vi "VisionV3 2-7-20.vi"(7 "error in":errorcluster, 10 "Image In":T2) -> (0 "error out":errorcluster, 1 "Number of Matches":i32, 2 "Shape Report":T1(array[cluster]) {"Score" format="%.2f"; "Centroid"."y" format="%.2f"; "Centroid"."x" format="%.2f"}, 3 "Image Out":T2)   [LabVIEW 2019]
uses:
  <vilib>/vision/Image Controls.llb/IMAQ Image.ctl
  <vilib>/vision/NI_Vision_Development_Module.lvlib
panel:
  out "Histogram (Histogram 1)":u32[][](array[numeric])
  out "Histogram Graph":u32[][](graph)
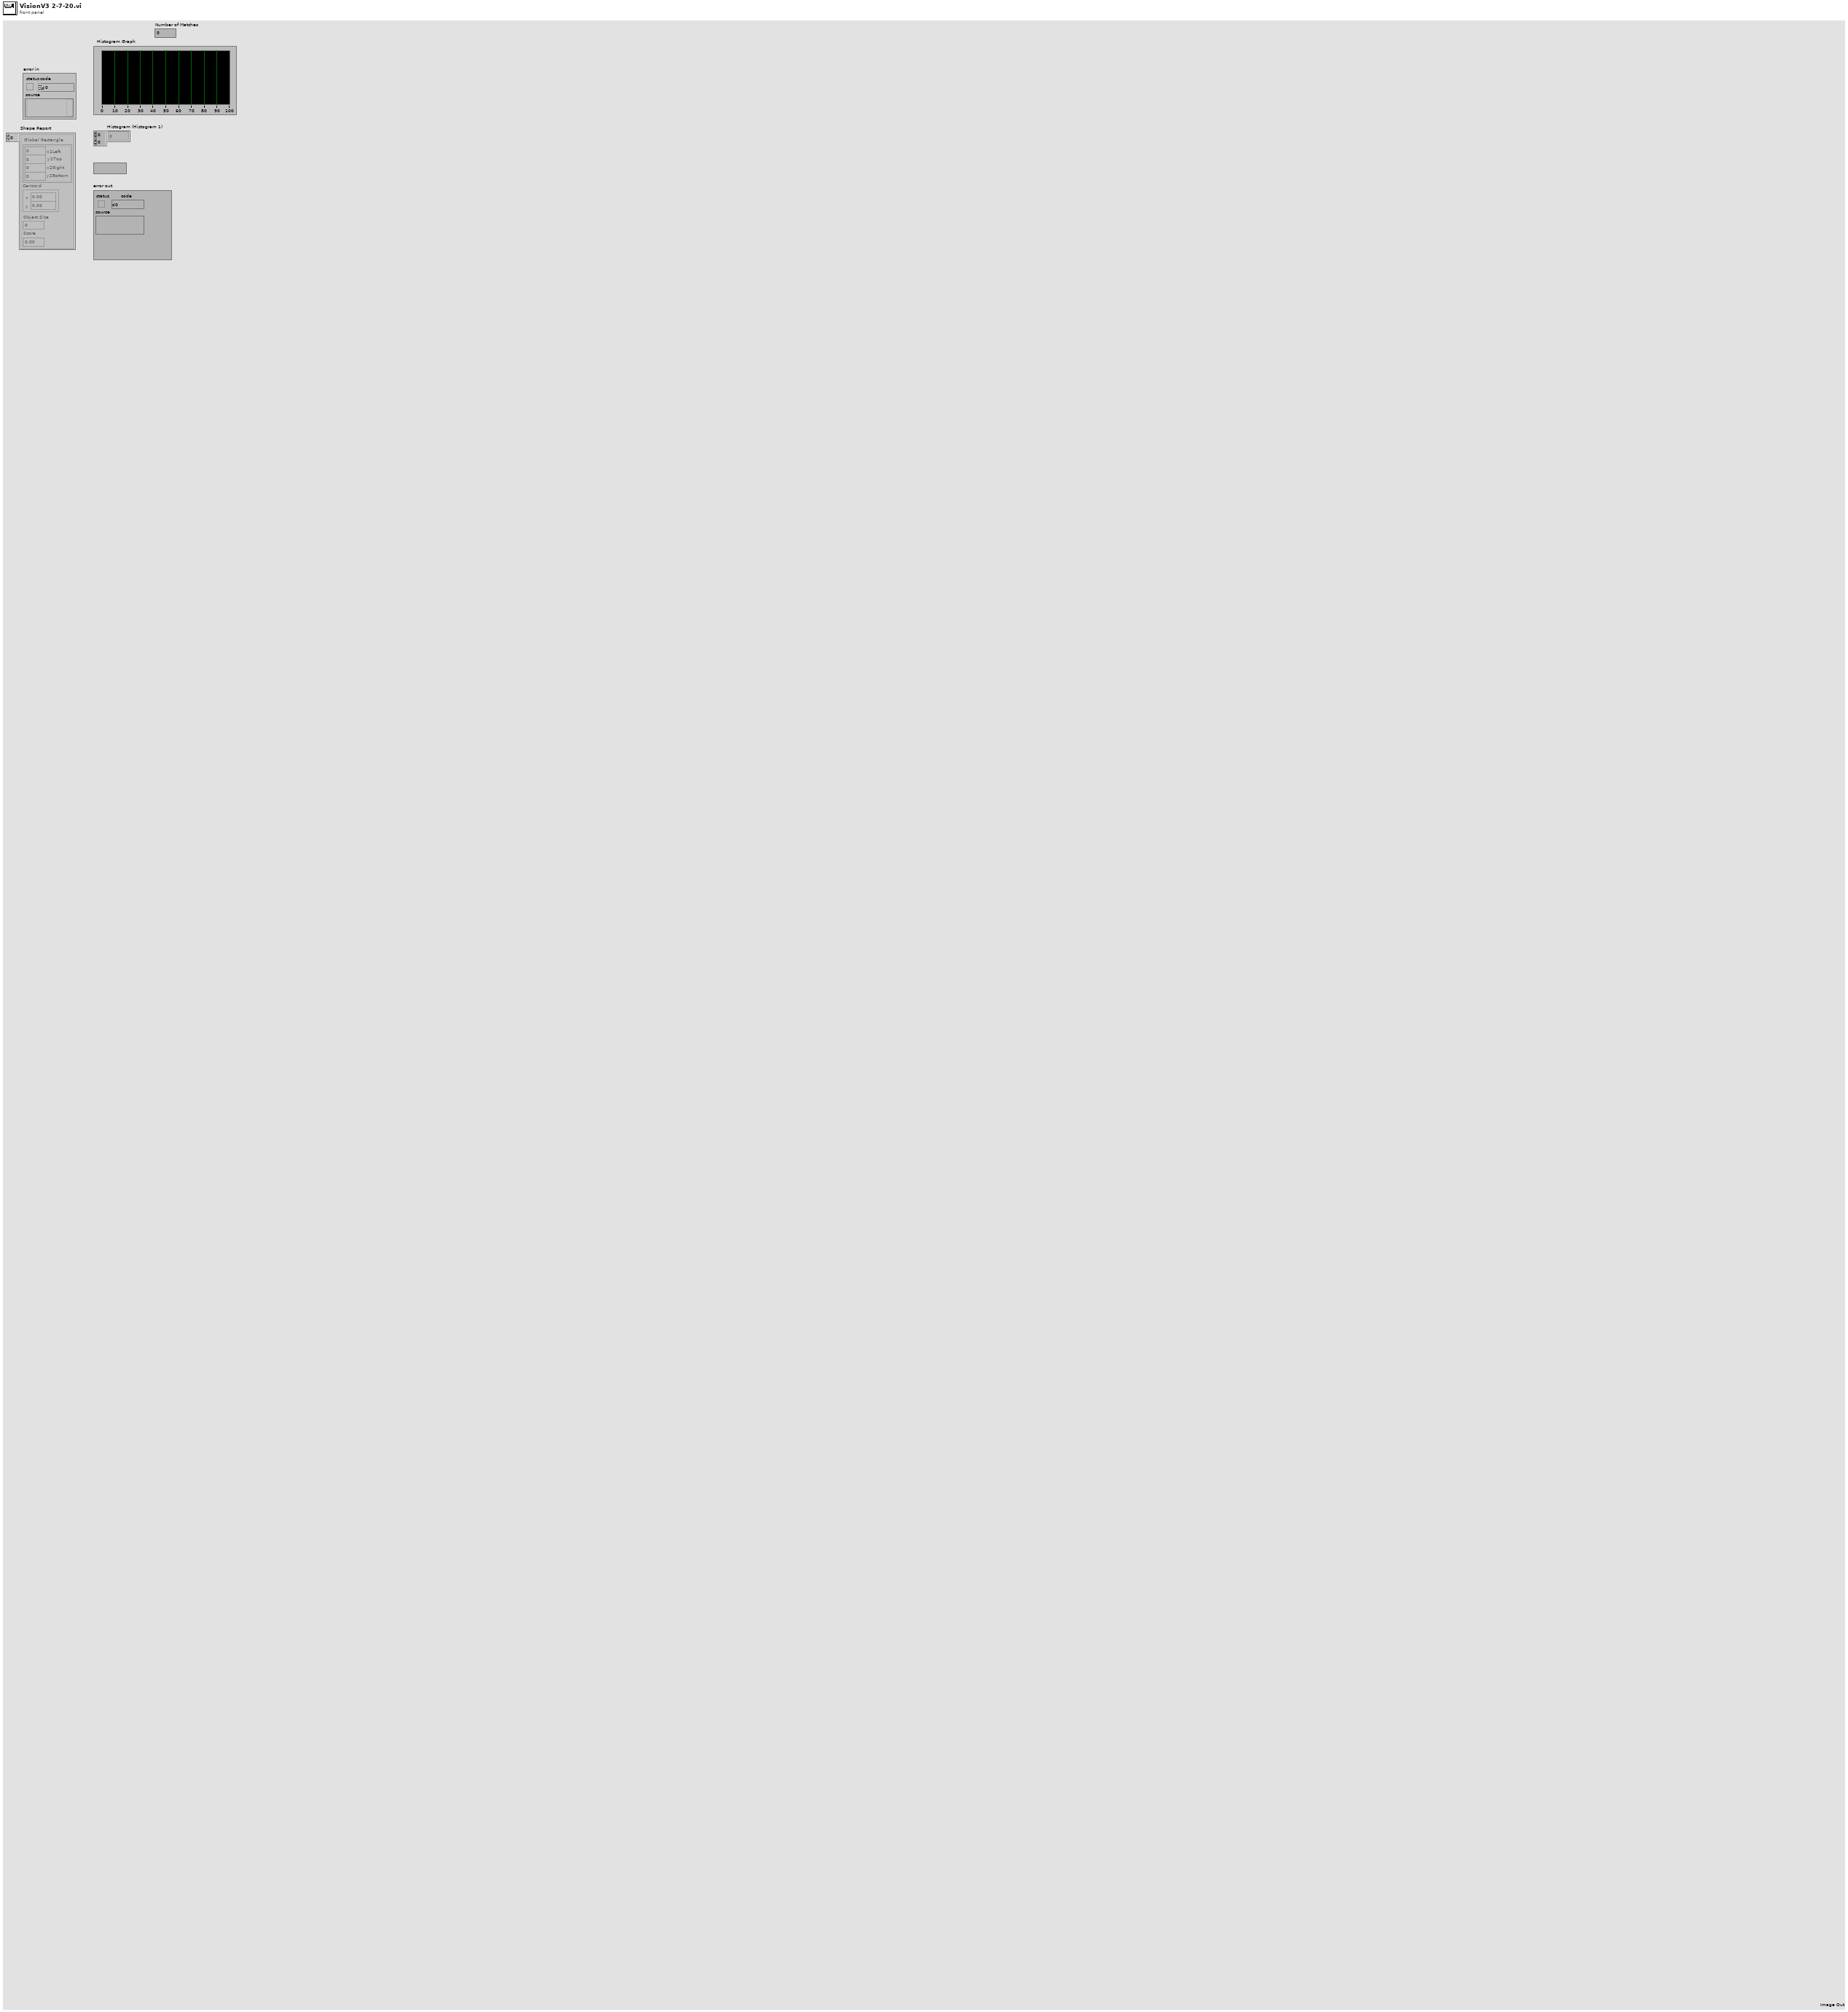
[diagram p1: front panel]
types:
  T1 = cluster{"Global Rectangle":cluster{"x1Left":i32, "y1Top":i32, "x2Right":i32, "y2Bottom":i32}, "Centroid":cluster{"x":sgl, "y":sgl}, "Object Size":u32, "Score":dbl}[]
  T2 = typedef "IMAQ Image.ctl" = refnum<image>
  T3 = enum32{"AutoM", "Close", "Dilate", "Erode", "Gradient", "Gradient in", "Gradient out", "HitMiss", "Open", "PClose", "POpen", "Thick", "Thin"}
  T4 = cluster{"Global Rectangle":i32[], "Contours":cluster{"ID":enum32{"External", "Internal"}, "Type":u32, "Coordinates":i32[]}[]}
  T5 = cluster{"histogram":u32[], "Minimal Value":sgl, "Maximal Value":sgl, "Starting Value":sgl, "Interval Width":sgl, "Mean Value":sgl, "Standard  Variation":sgl, "Area (pixels)":i32}
  T6 = typedef "Image Type" = u32
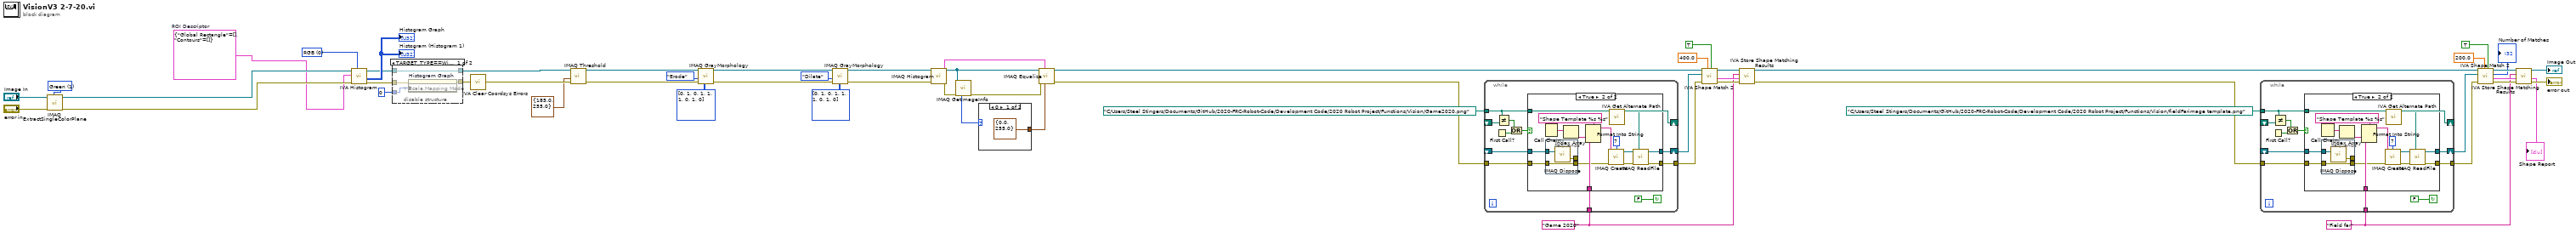
[diagram p0: block diagram]
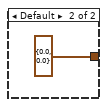
[diagram p4: hidden frame]
diagram:
  w2 = "Field far" ("Step Name")
  w14 = "Game 2020" ("Step Name")
  w49 = u16 0 items=["RGB", "HSL", "HSV", "HSI"] ("Color Mode")
  w47 = T4 {"Global Rectangle"=[], "Contours"=[]}  # ROI Descriptor
  w55 = 1 items=["Red", "Green", "Blue", "Hue", "Saturation", "Luminance", "Value", "Intensity"] ("Color Plane")
  n1 = call "IMAQ ExtractSingleColorPlane"("Color Plane"=w55, "error in (no error)"="error in", "Image Src"="Image In") -> ("error out"=w52:errorcluster, "Image Dst Out"=w51:T2)  [unwired: 1 in, 6 out]
  n2 = call <vilib>:"IVA Histogram.vi"("Color Mode"=w49, "error in (no error)"=w52, "ROI Descriptor"=w47, "Image In"=w51) -> ("error out"=w50:errorcluster, "Histograms"=→"Histogram Graph" →"Histogram (Histogram 1)":u32[][], "Image Out"=w46:T2)  [unwired: 5 out]
  n3 = disable-structure "Conditional Disable Structure" shown="TARGET_TYPE==Windows" {
    disable-tunnel: w50 -> [w59 w60]
    disable-tunnel: [w58 w60] -> w44
    disable-tunnel: w46 -> [w57 w61]
    disable-tunnel: [w57 w61] -> w41
    disable-tunnel: u8 0 ("Y Scale.Mapping Mode") -> [w56 _]
    frame condition #0 {
      n4 = property on="Histogram Graph" class="WFGraph (strict)"(error in=w59, "Y Scale.Mapping Mode"=w56) -> (error out=w58:errorcluster)  [unwired: 1 in, 1 out]
    }
    frame condition #1 (active) {
    }
  }
  n5 = call <vilib>:"IVA Clear Coordsys Errors.vi"("error in (no error)"=w44) -> ("error out"=w43:errorcluster)  [unwired: 10 in]
  n6 = call "IMAQ Threshold"("error in (no error)"=w43, "Range"=cluster{"Lower value":sgl, "Upper value":sgl} {"Lower value"=185.0, "Upper value"=255.0}, "Image Src"=w41) -> ("error out"=w40:errorcluster, "Image Dst Out"=w37:T2)  [unwired: 3 in, 4 out]
  n7 = call "IMAQ GrayMorphology"("Structuring Element"=i32[][] [[0, 1, 0], [1, 1, 1], [0, 1, 0]], "error in (no error)"=w40, "Operation"=T3."Erode", "Image Src"=w37) -> ("error out"=w36:errorcluster, "Image Dst Out"=w33:T2)  [unwired: 3 in, 3 out]
  n8 = call "IMAQ GrayMorphology"("Structuring Element"=i32[][] [[0, 1, 0], [1, 1, 1], [0, 1, 0]], "error in (no error)"=w36, "Operation"=T3."Dilate", "Image Src"=w33) -> ("error out"=w32:errorcluster, "Image Dst Out"=w28:T2)  [unwired: 3 in, 3 out]
  n9 = call "IMAQ Histogram"("error in (no error)"=w32, "Image"=w28) -> ("error out"=w27:errorcluster, "Histogram Report"=w30:T5)  [unwired: 3 in, 5 out]
  n10 = call "IMAQ GetImageInfo"("error in (no error)"=w27, "Image"=w28) -> ("error out"=w26:errorcluster, "Image Type"=w29:T6)  [unwired: 8 out]
  n11 = case shown="0" w29 {
    tunnel: [cluster{"Minimum":sgl, "Maximum":sgl} {"Minimum"=0.0, "Maximum"=255.0} ("Range") cluster{"Minimum":sgl, "Maximum":sgl} {"Minimum"=0.0, "Maximum"=0.0} ("Range")] -> w25
    frame 0 {
    }
    frame Default {
    }
  }
  n12 = call "IMAQ Equalize"("Range"=w25, "Histogram Report"=w30, "error in (no error)"=w26, "Image Src"=w28) -> ("error out"=w31:errorcluster, "Image Dst Out"=w22:T2)  [unwired: 2 in, 4 out]
  n13 = while {
    shift-right: [w74] -> w15
    shift-left: _ -> [w73]
    tunnel: [w71] -> w16
    tunnel: w31 -> [w70]
    tunnel: path "C:/Users/Steel Stingers/Documents/GitHub/2020-FRC-Robot-Code/Development Code/2020 Robot Project/Functions/Vision/Game2020.png" ("Template Path") -> [w68]
    tunnel: w14 -> [w69]
    shift-right: [w68] -> _
    shift-left: _ -> [w67]
    stop <- FALSE continue-if-true
    n14 = First Call?() -> (First Call?: T/F=w66:bool)
    n15 = Not Equal?(x=w68, y=w67) -> (x != y?=w65:bool)
    n16 = Or(x=w65, y=w66) -> (x .or. y?=w64:bool)
    n17 = case shown="True" w64 {
      tunnel: [w76 w88] -> w74
      tunnel: w73 -> [w76 w79]
      tunnel: [w75 w86] -> w71
      tunnel: w70 -> [w75 w78]
      tunnel: w68 -> [_ w81]
      tunnel: w69 -> [_ w82]
      frame False {
      }
      frame True {
        n18 = Call Chain() -> (call chain=w84:string[])
        n19 = stacked-sequence {
          tunnel: w79 -> [w94]
          tunnel: w78 -> [w93]
          tunnel: [w93] -> w77
          tunnel: [w92] -> _
          frame #0 {
            n20 = call "IMAQ Dispose"("Image"=w94) -> ("error out"=w92:errorcluster)  [unwired: 2 in, 3 out]
          }
        }
        n21 = Index Array(array=w84) -> (element=w83:string)  [unwired: 1 in]
        n22 = Format Into String(format string="Shape Template %s %s" ("Image Name"), w83, w82) -> (resulting string=w91:string)  [unwired: 2 in, 1 out]
        n23 = call "IMAQ Create"("Border Size"=7, "Image Name"=w91, "error in (no error)"=w77) -> ("New Image"=w89:T2, "error out"=w87:errorcluster)  [unwired: 1 in, 1 out]
        n24 = call <vilib>:"IVA Get Alternate Path.vi"("Path In"=w81) -> ("Path Out"=w80:path)  [unwired: 10 out]
        n25 = call "IMAQ ReadFile"("File Path"=w80, "error in (no error)"=w87, "Image"=w89) -> ("error out"=w86:errorcluster, "Image Out"=w88:T2)  [unwired: 2 in, 5 out]
      }
    }
  }
  n26 = call <vilib>:"IVA Shape Match 2.vi"("Scale Invariance"=TRUE, "Minimal Score"=400.0, "error in (no error)"=w16, "Template"=w15, "Image Src"=w22) -> ("error out"=w21:errorcluster, "Shape Report"=w19:T1, "Image Out"=w18:T2)  [unwired: 4 out]
  n27 = call <vilib>:"IVA Store Shape Matching Results.vi"("error in (no error)"=w21, "Shape Report"=w19, "Step Name"=w14, "Image in"=w18) -> ("error out"=w20:errorcluster, "Image dup"=w11:T2)  [unwired: 6 out]
  n28 = while {
    shift-right: [w105] -> w3
    shift-left: _ -> [w104]
    tunnel: [w102] -> w4
    tunnel: w20 -> [w101]
    tunnel: path "C:/Users/Steel Stingers/Documents/GitHub/2020-FRC-Robot-Code/Development Code/2020 Robot Project/Functions/Vision/fieldFarimage template.png" ("Template Path") -> [w99]
    tunnel: w2 -> [w100]
    shift-right: [w99] -> _
    shift-left: _ -> [w98]
    stop <- FALSE continue-if-true
    n29 = First Call?() -> (First Call?: T/F=w97:bool)
    n30 = Not Equal?(x=w99, y=w98) -> (x != y?=w96:bool)
    n31 = Or(x=w96, y=w97) -> (x .or. y?=w95:bool)
    n32 = case shown="True" w95 {
      tunnel: [w107 w119] -> w105
      tunnel: w104 -> [w107 w110]
      tunnel: [w106 w117] -> w102
      tunnel: w101 -> [w106 w109]
      tunnel: w99 -> [_ w112]
      tunnel: w100 -> [_ w113]
      frame False {
      }
      frame True {
        n33 = Call Chain() -> (call chain=w115:string[])
        n34 = stacked-sequence {
          tunnel: w110 -> [w125]
          tunnel: w109 -> [w124]
          tunnel: [w124] -> w108
          tunnel: [w123] -> _
          frame #0 {
            n35 = call "IMAQ Dispose"("Image"=w125) -> ("error out"=w123:errorcluster)  [unwired: 2 in, 3 out]
          }
        }
        n36 = Index Array(array=w115) -> (element=w114:string)  [unwired: 1 in]
        n37 = Format Into String(format string="Shape Template %s %s" ("Image Name"), w114, w113) -> (resulting string=w122:string)  [unwired: 2 in, 1 out]
        n38 = call "IMAQ Create"("Border Size"=7, "Image Name"=w122, "error in (no error)"=w108) -> ("New Image"=w120:T2, "error out"=w118:errorcluster)  [unwired: 1 in, 1 out]
        n39 = call <vilib>:"IVA Get Alternate Path.vi"("Path In"=w112) -> ("Path Out"=w111:path)  [unwired: 10 out]
        n40 = call "IMAQ ReadFile"("File Path"=w111, "error in (no error)"=w118, "Image"=w120) -> ("error out"=w117:errorcluster, "Image Out"=w119:T2)  [unwired: 2 in, 5 out]
      }
    }
  }
  n41 = call <vilib>:"IVA Shape Match 2.vi"("Scale Invariance"=TRUE, "Minimal Score"=200.0, "error in (no error)"=w4, "Template"=w3, "Image Src"=w11) -> ("error out"=w10:errorcluster, "Shape Report"=w8:T1, "Number of Matches"=→"Number of Matches":i32, "Image Out"=w7:T2)  [unwired: 3 out]
  "Shape Report" <- w8
  n42 = call <vilib>:"IVA Store Shape Matching Results.vi"("error in (no error)"=w10, "Shape Report"=w8, "Step Name"=w2, "Image in"=w7) -> ("error out"=→"error out":errorcluster, "Image dup"=→"Image Out":T2)  [unwired: 6 out]
